vi "State Machine Fail Check.vi"() -> ()   [LabVIEW 2022 SP3]
panel:
  in  "Fail Check":bool
  # "Intialization\ntemprature control\nPressure Control\nFail Check\nFail State"
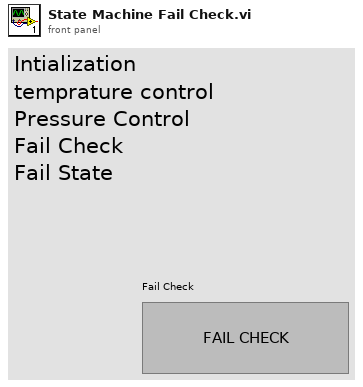
[diagram p1: front panel]
types:
  T1 = enum16{"Intialization", "Temprature Control", "Pressure Control", "Fail Check", "Fail State"}
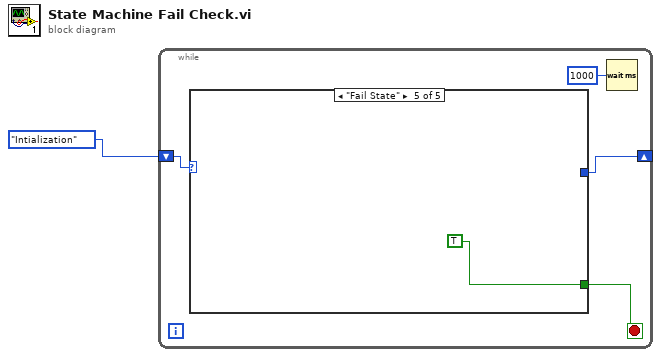
[diagram p0: block diagram]
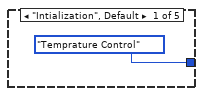
[diagram p2: hidden frame]
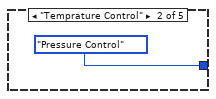
[diagram p3: hidden frame]
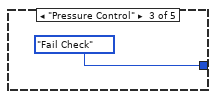
[diagram p4: hidden frame]
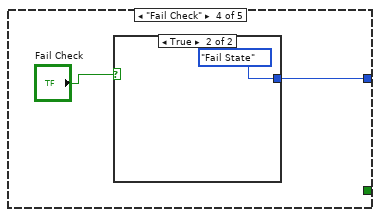
[diagram p5: hidden frame]
diagram:
  n1 = while {
    shift-right: [w4] -> _
    shift-left: T1."Intialization" -> [w5]
    stop <- w3 stop-if-true
    n2 = case shown="\"Fail State\"" w5 {
      tunnel: [T1."Temprature Control" T1."Pressure Control" T1."Fail Check" w10 _] -> w4
      tunnel: [_ _ _ _ TRUE] -> w3
      frame "Intialization", Default {
      }
      frame "Temprature Control" {
      }
      frame "Pressure Control" {
      }
      frame "Fail Check" {
        n3 = case shown="True" "Fail Check" {
          tunnel: [_ T1."Fail State"] -> w10
          frame False {
          }
          frame True {
          }
        }
      }
      frame "Fail State" {
      }
    }
    n4 = Wait (ms)(milliseconds to wait=u32 1000) -> ()  [unwired: 1 out]
  }
